vi "Repack Pixels_FIFO to Pixel Bus HSL32x8.vi"(8 "Last \npacket length":u8, 9 "Last valid \npacket - Image":bool, 10 "Last valid \npacket - Row":bool, 11 "Source Image FIFO":refnum<k21>) -> (1 "Read/No Read":bool, 2 "DV Out":bool, 3 "Pixel Bus Out":T1={"Pixel Data"={"A"=[0, 0, 0, 0, 0, 0, 0, 0], "R/H"=[0, 0, 0, 0, 0, 0, 0, 0], "G/S"=[0, 0, 0, 0, 0, 0, 0, 0], "B/L"=[0, 0, 0, 0, 0, 0, 0, 0]}, "DV"=[FALSE, FALSE, FALSE, FALSE, FALSE, FALSE, FALSE, FALSE], "EOL"=FALSE, "EOI"=FALSE, "Data Type"=enum."HSL32 x 8"})   [LabVIEW 2020, in "NI_VDM_FPGA_Basics.lvlib"]
uses:
  <vilib>/visionFPGA/NI_VDM_FPGA_Basics.lvlib
  <vilib>/visionFPGA/Controls/IMAQ FPGA Pixel Bus HSL32x8.ctl
  <vilib>/rvi/DataTransferAndStorage/Container/XNode/niFpgaContainer.xnode
  <vilib>/rvi/FIFO/Fifo_Resource/niFpgaFifoEmulationRefInMultiElement.vi
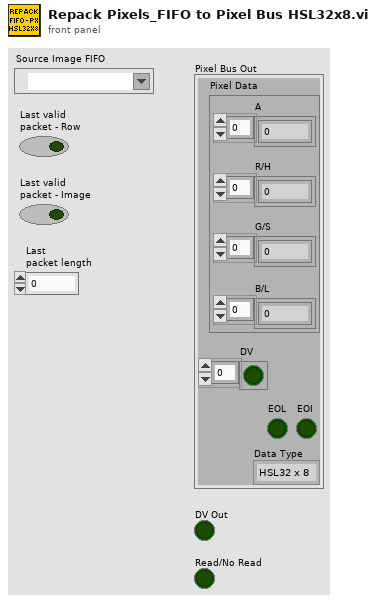
[diagram p1: front panel]
types:
  T1 = typedef "IMAQ FPGA Pixel Bus HSL32x8.ctl" = cluster{"Pixel Data":cluster{"A":u8[], "R/H":u8[], "G/S":u8[], "B/L":u8[]}, "DV":bool[], "EOL":bool, "EOI":bool, "Data Type":enum16{"HSL32 x 8"}}
  T2 = cluster{"A":u8[], "R/H":u8[], "G/S":u8[], "B/L":u8[]}
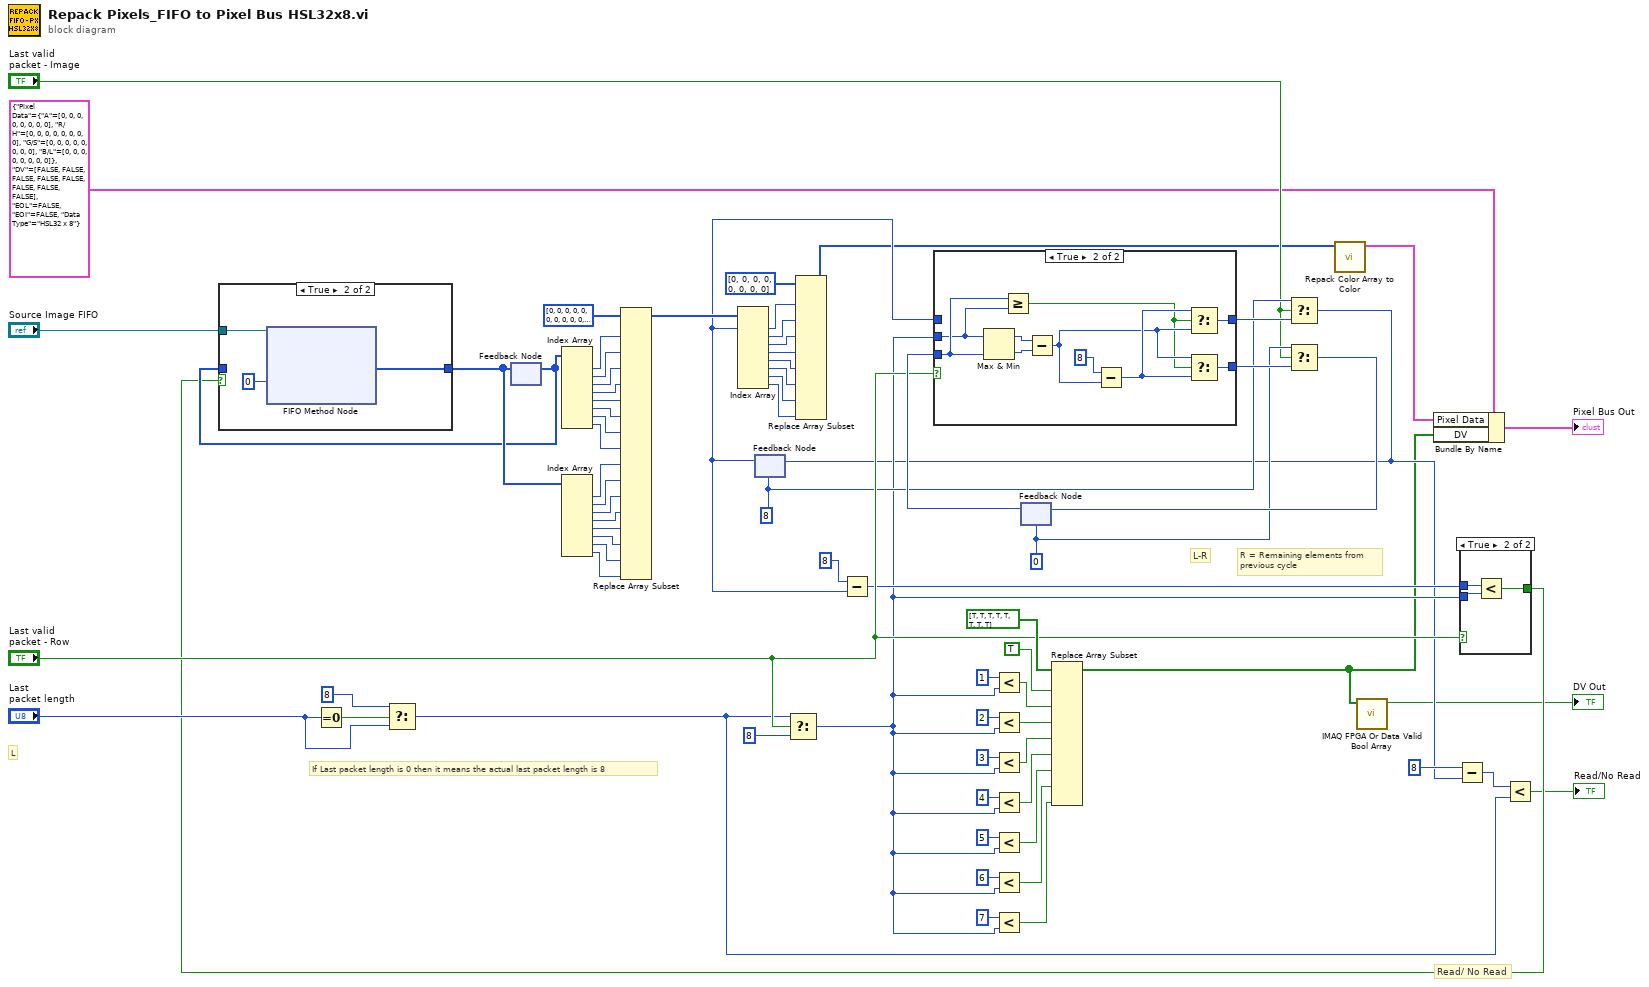
[diagram p0: block diagram]
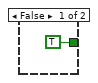
[diagram p3: hidden frame]
diagram:
  w16 = u8 0
  w17 = u8 8
  # "L"
  # "L-R"
  # "If Last packet length is 0 then it means the actual last packet length is 8"
  # "Read/ No Read"
  # "R = Remaining elements from\nprevious cycle"
  n1 = Equal To 0?(x="Last \npacket length") -> (x = 0?=w36:bool)
  n2 = Select(t=u8 8, s=w36, f="Last \npacket length") -> (s? t:f=w5:u8)
  n3 = feedback #1() -> (w22:u32[])  [unwired: 1 in]
  n4 = Index Array(array=w22) -> (element #1=w55:u32, element #2=w54:u32, element #3=w53:u32, element #4=w52:u32, element #5=w51:u32, element #6=w50:u32, element #7=w49:u32, element #8=w48:u32)  [unwired: 8 in]
  n5 = feedback #2(w17) -> (w13:u8)
  n6 = Select(t=w5, s="Last valid \npacket - Row", f=u8 8) -> (s? t:f=w10:u8)
  n7 = Subtract(x=u8 8, y=w13) -> (x-y=w11:u8)
  n8 = Less?(x=u8 1, y=w10) -> (x < y?=w62:bool)
  n9 = Less?(x=u8 2, y=w10) -> (x < y?=w61:bool)
  n10 = Less?(x=u8 3, y=w10) -> (x < y?=w60:bool)
  n11 = Less?(x=u8 4, y=w10) -> (x < y?=w59:bool)
  n12 = Less?(x=u8 5, y=w10) -> (x < y?=w58:bool)
  n13 = Less?(x=u8 6, y=w10) -> (x < y?=w57:bool)
  n14 = Less?(x=u8 7, y=w10) -> (x < y?=w56:bool)
  n15 = feedback #3(w16) -> (w24:u8)
  n16 = case shown="True" "Last valid \npacket - Row" {
    tunnel: w24 -> [w75 w86]
    tunnel: w10 -> [_ w85]
    tunnel: [w76 w84] -> w19
    tunnel: [w75 w83] -> w18
    tunnel: w13 -> [w76 _]
    frame False {
    }
    frame True {
      n17 = Max & Min(x=w85, y=w86) -> (max(x,y)=w80:u8, min(x,y)=w79:u8)
      n18 = Greater Or Equal?(x=w86, y=w85) -> (x >= y?=w77:bool)
      n19 = Subtract(x=w80, y=w79) -> (x-y=w81:u8)
      n20 = Subtract(x=u8 8, y=w81) -> (x-y=w82:u8)
      n21 = Select(t=w82, s=w77, f=w81) -> (s? t:f=w84:u8)
      n22 = Select(t=w81, s=w77, f=w82) -> (s? t:f=w83:u8)
    }
  }
  n23 = Replace Array Subset(array=bool[] [TRUE, TRUE, TRUE, TRUE, TRUE, TRUE, TRUE, TRUE], new element #1=TRUE ("new element/subarray"), new element #2=w62, new element #3=w61, new element #4=w60, new element #5=w59, new element #6=w58, new element #7=w57, new element #8=w56) -> (w2:bool[])  [unwired: 8 in]
  n24 = Select(t=w17, s="Last valid \npacket - Image", f=w19) -> (s? t:f=w8:u8)
  n25 = feedback-in #2(w8) -> ()
  n26 = Select(t=w16, s="Last valid \npacket - Image", f=w18) -> (s? t:f=w20:u8)
  n27 = feedback-in #3(w20) -> ()
  n28 = call <vilib>:"IMAQ FPGA Or Data Valid Bool Array.vi"("DV Array In"=w2) -> ("DV Out"=→"DV Out":bool)  [unwired: 10 in]
  n29 = Subtract(x=u8 8, y=w8) -> (x-y=w7:u8)
  n30 = case shown="True" "Last valid \npacket - Row" {
    tunnel: w10 -> [_ w89]
    tunnel: w11 -> [_ w90]
    tunnel: [TRUE w88] -> w12
    frame False {
    }
    frame True {
      n31 = Less?(x=w90, y=w89) -> (x < y?=w88:bool)
    }
  }
  n32 = case shown="True" w12 {
    tunnel: "Source Image FIFO" -> [_ w94]
    tunnel: [w91 w92] -> w47
    tunnel: w22 -> [w91 _]
    frame False {
    }
    frame True {
      n33 = xnode ("FIFO Method Node")("Timeout"=0, "FIFO In"=w94) -> ("Element"=w92:u32[])  [unwired: 2 out]
    }
  }
  n34 = feedback-in #1(w47) -> ()
  n35 = Index Array(array=w47) -> (element #1=w46:u32, element #2=w45:u32, element #3=w44:u32, element #4=w43:u32, element #5=w42:u32, element #6=w41:u32, element #7=w40:u32, element #8=w39:u32)  [unwired: 8 in]
  n36 = Replace Array Subset(array=u32[] [0, 0, 0, 0, 0, 0, 0, 0, 0, 0, 0, 0, 0, 0, 0, 0], new element #1=w55, new element #2=w54, new element #3=w53, new element #4=w52, new element #5=w51, new element #6=w50, new element #7=w49, new element #8=w48, new element #9=w46, new element #10=w45, new element #11=w44, new element #12=w43, new element #13=w42, new element #14=w41, new element #15=w40, new element #16=w39) -> (w23:u32[])  [unwired: 16 in]
  n37 = Index Array(array=w23, index #1=w13) -> (element #1=w33:u32, element #2=w32:u32, element #3=w31:u32, element #4=w30:u32, element #5=w29:u32, element #6=w28:u32, element #7=w27:u32, element #8=w26:u32)  [unwired: 7 in]
  n38 = Replace Array Subset(array=u32[] [0, 0, 0, 0, 0, 0, 0, 0], new element #1=w33, new element #2=w32, new element #3=w31, new element #4=w30, new element #5=w29, new element #6=w28, new element #7=w27, new element #8=w26) -> (w3:u32[])  [unwired: 8 in]
  n39 = call <vilib>:"Repack Color Array to Color.vi"("Input Array U32x8"=w3) -> ("Colour Pixel Data"=w4:T2)  [unwired: 10 in]
  n40 = Bundle By Name(cluster=T1 {"Pixel Data"={"A"=[0, 0, 0, 0, 0, 0, 0, 0], "R/H"=[0, 0, 0, 0, 0, 0, 0, 0], "G/S"=[0, 0, 0, 0, 0, 0, 0, 0], "B/L"=[0, 0, 0, 0, 0, 0, 0, 0]}, "DV"=[FALSE, FALSE, FALSE, FALSE, FALSE, FALSE, FALSE, FALSE], "EOL"=FALSE, "EOI"=FALSE, "Data Type"=enum."HSL32 x 8"} ("Pixel Bus Out 2"), "Pixel Data"=w4, "DV"=w2) -> (→"Pixel Bus Out":T1)
  n41 = Less?(x=w7, y=w5) -> (x < y?=→"Read/No Read":bool)
